vi "MoveOffLimit.vi"(8 "error in (no error)":errorcluster, 10 "controllerAddress":i32, 11 "reference":refnum<k24>) -> (0 "error out":errorcluster, 2 "controllerAddress out":i32, 3 "reference out":refnum<k24>)   [LabVIEW 2013]
uses:
  C:/Program Files/Newport/Piezo Motion Control/Newport AG-UC2-UC8 Applet/Samples/LabVIEW 2009/AgilisCmdLib.dll
  Program Files/Newport/Piezo Motion Control/Newport AG-UC2-UC8 Applet/Samples/LabVIEW 2009/AgilisCmdLib.dll
panel:
  out "LimitStatus 2":i32
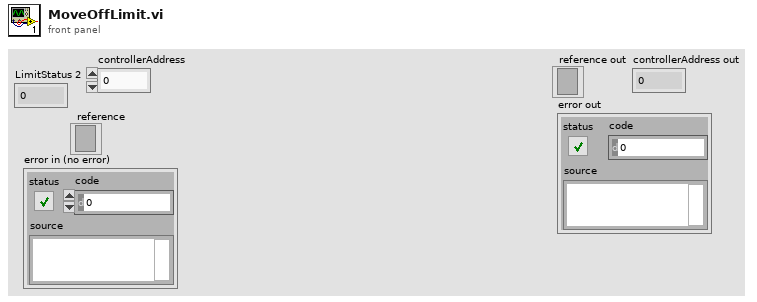
[diagram p1: front panel]
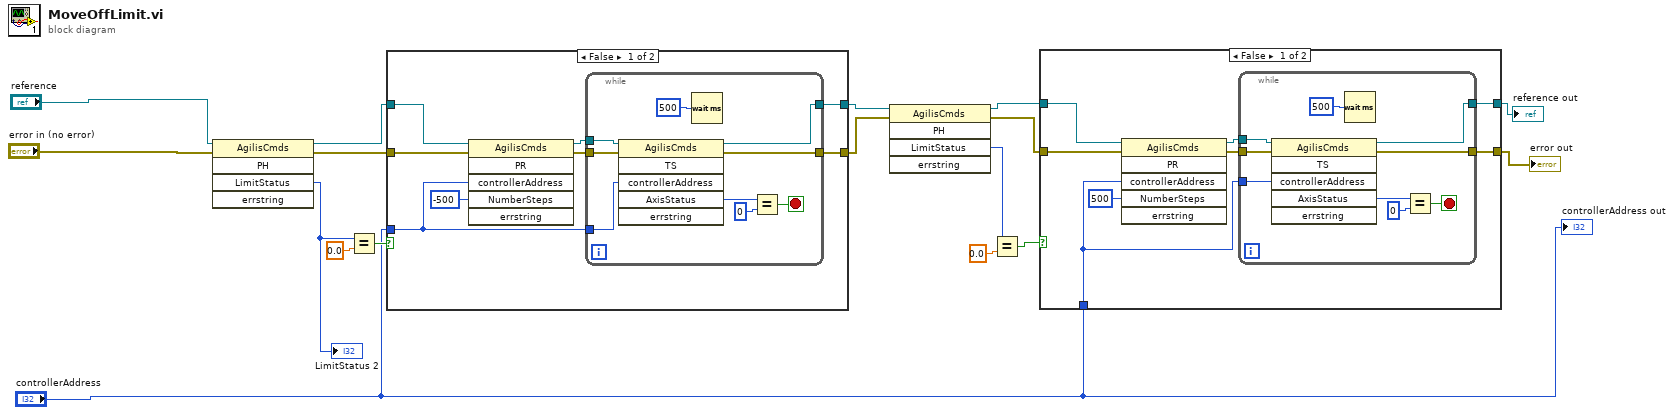
[diagram p0: block diagram]
diagram:
  n1 = invoke class="AgilisCmds" method="PH"(reference="reference", error in="error in (no error)") -> (reference out=w11:refnum<k24>, error out=w15:errorcluster, "LimitStatus"=w14:i32)  [unwired: 3 in, 2 out]
  "LimitStatus 2" <- w14
  n2 = Equal?(x=w14, y=0.0) -> (x = y?=w12:bool)
  n3 = case shown="False" w12 {
    tunnel: w15 -> [w23 w36]
    tunnel: [w22 w35] -> w9
    tunnel: [w21 w36] -> w8
    tunnel: w11 -> [w20 w35]
    tunnel: "controllerAddress" -> [w19 _]
    frame False {
      n4 = invoke class="AgilisCmds" method="PR"(reference=w20, error in=w23, "controllerAddress"=w19, "NumberSteps"=i64 -500) -> (reference out=w25:refnum<k24>, error out=w24:errorcluster)  [unwired: 2 in, 4 out]
      n5 = while {
        tunnel: [w34] -> w21
        tunnel: w25 -> [w29]
        tunnel: w24 -> [w28]
        tunnel: [w27] -> w22
        tunnel: w19 -> [w26]
        stop <- w31 stop-if-true
        n6 = invoke class="AgilisCmds" method="TS"(reference=w29, error in=w28, "controllerAddress"=w26) -> (reference out=w27:refnum<k24>, error out=w34:errorcluster, "AxisStatus"=w33:i32)  [unwired: 3 in, 3 out]
        n7 = Wait (ms)(milliseconds to wait=u32 500) -> ()  [unwired: 1 out]
        n8 = Equal?(x=w33, y=0) -> (x = y?=w31:bool)
      }
    }
    frame True {
    }
  }
  n9 = invoke class="AgilisCmds" method="PH"(reference=w9, error in=w8) -> (reference out=w7:refnum<k24>, error out=w6:errorcluster, "LimitStatus"=w5:i32)  [unwired: 3 in, 2 out]
  n10 = Equal?(x=w5, y=0.0) -> (x = y?=w4:bool)
  n11 = case shown="False" w4 {
    tunnel: w6 -> [w42 w55]
    tunnel: [w41 w54] -> w3
    tunnel: [w40 w55] -> w2
    tunnel: w7 -> [w39 w54]
    tunnel: "controllerAddress" -> [w37 _]
    frame False {
      n12 = invoke class="AgilisCmds" method="PR"(reference=w39, error in=w42, "controllerAddress"=w37, "NumberSteps"=i64 500) -> (reference out=w44:refnum<k24>, error out=w43:errorcluster)  [unwired: 2 in, 4 out]
      n13 = while {
        tunnel: [w53] -> w40
        tunnel: w44 -> [w48]
        tunnel: w43 -> [w47]
        tunnel: [w46] -> w41
        tunnel: w37 -> [w45]
        stop <- w50 stop-if-true
        n14 = invoke class="AgilisCmds" method="TS"(reference=w48, error in=w47, "controllerAddress"=w45) -> (reference out=w46:refnum<k24>, error out=w53:errorcluster, "AxisStatus"=w52:i32)  [unwired: 3 in, 3 out]
        n15 = Wait (ms)(milliseconds to wait=u32 500) -> ()  [unwired: 1 out]
        n16 = Equal?(x=w52, y=0) -> (x = y?=w50:bool)
      }
    }
    frame True {
    }
  }
  "error out" <- w2
  "reference out" <- w3
  "controllerAddress out" <- "controllerAddress"
